vi "Generate Pixel Pulse.vi"(10 "Ready For Output":bool, 11 "Data":u32) -> (2 "Done":bool, 3 "Pulse Output":bool)   [LabVIEW 2021, in "Neopixel - FPGA.lvclass"]
uses:
  Neopixel - FPGA.lvclass
  Neopixel - FPGA.lvclass/Neopixel - FPGA.ctl
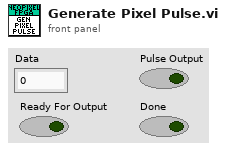
[diagram p1: front panel]
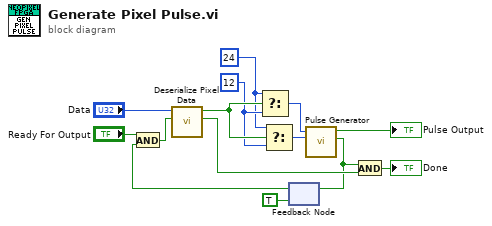
[diagram p0: block diagram]
diagram:
  w5 = u8 12 ("High False")
  w4 = u8 24 ("High True")
  n1 = feedback #1(TRUE ("Ready For Input")) -> (w1:bool)
  n2 = And(x="Ready For Output", y=w1) -> (x .and. y?=w2:bool)
  n3 = call "Deserialize Pixel Data.vi"("Ready For Output"=w2, "Data"="Data") -> ("Done"=w12:bool, "Value"=w9:bool)  [unwired: 8 in]
  n4 = Select(t=w4, s=w9, f=w5) -> (s? t:f=w7:u8)
  n5 = Select(t=w4, s=w9, f=w5) -> (s? t:f=w8:u8)
  n6 = call "Pulse Generator.vi"("Time Low (Ticks)"=w8, "Time High (Ticks)"=w7) -> ("Done"=w11:bool, "Pulse Output"=→"Pulse Output":bool)  [unwired: 8 in]
  n7 = feedback-in #1(w11) -> ()
  n8 = And(x=w11, y=w12) -> (x .and. y?=→"Done":bool)
